vi "Set Binary.vi"(8 "error in (no error)":errorcluster, 10 "Binary":bool, 11 "WebsocketStream in":refnum<class "WebsocketStream.lvclass">) -> (0 "error out":errorcluster, 3 "WebsocketStream out":refnum<class "WebsocketStream.lvclass">)   [LabVIEW 2020, in "Stream-Websocket.lvlib" / "WebsocketStream.lvclass"]
uses:
  WebsocketStream.lvclass
  WebsocketStream.lvclass/WebsocketStream.ctl
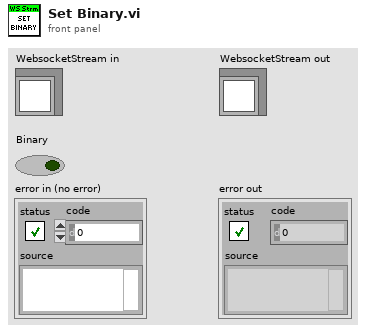
[diagram p1: front panel]
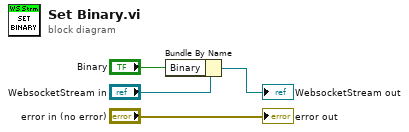
[diagram p0: block diagram]
diagram:
  n1 = Bundle By Name(cluster="WebsocketStream in", "Binary"="Binary") -> (→"WebsocketStream out":refnum<class "WebsocketStream.lvclass">)
  "error out" <- "error in (no error)"
